vi "Reset old test Values (SubVI).vi"(8 "error in":errorcluster, 9 "Atr in":refnum<vi>, 11 "Test Paragraph":string) -> (0 "error out":errorcluster, 1 "Atr out":refnum<vi>, 2 "Line number":i32, 3 "Atr Out":string[][](array[string]))   [LabVIEW 2017]
uses:
  <vilib>/Utility/miscctls.llb/LVRowAndColumnTypeDef.ctl
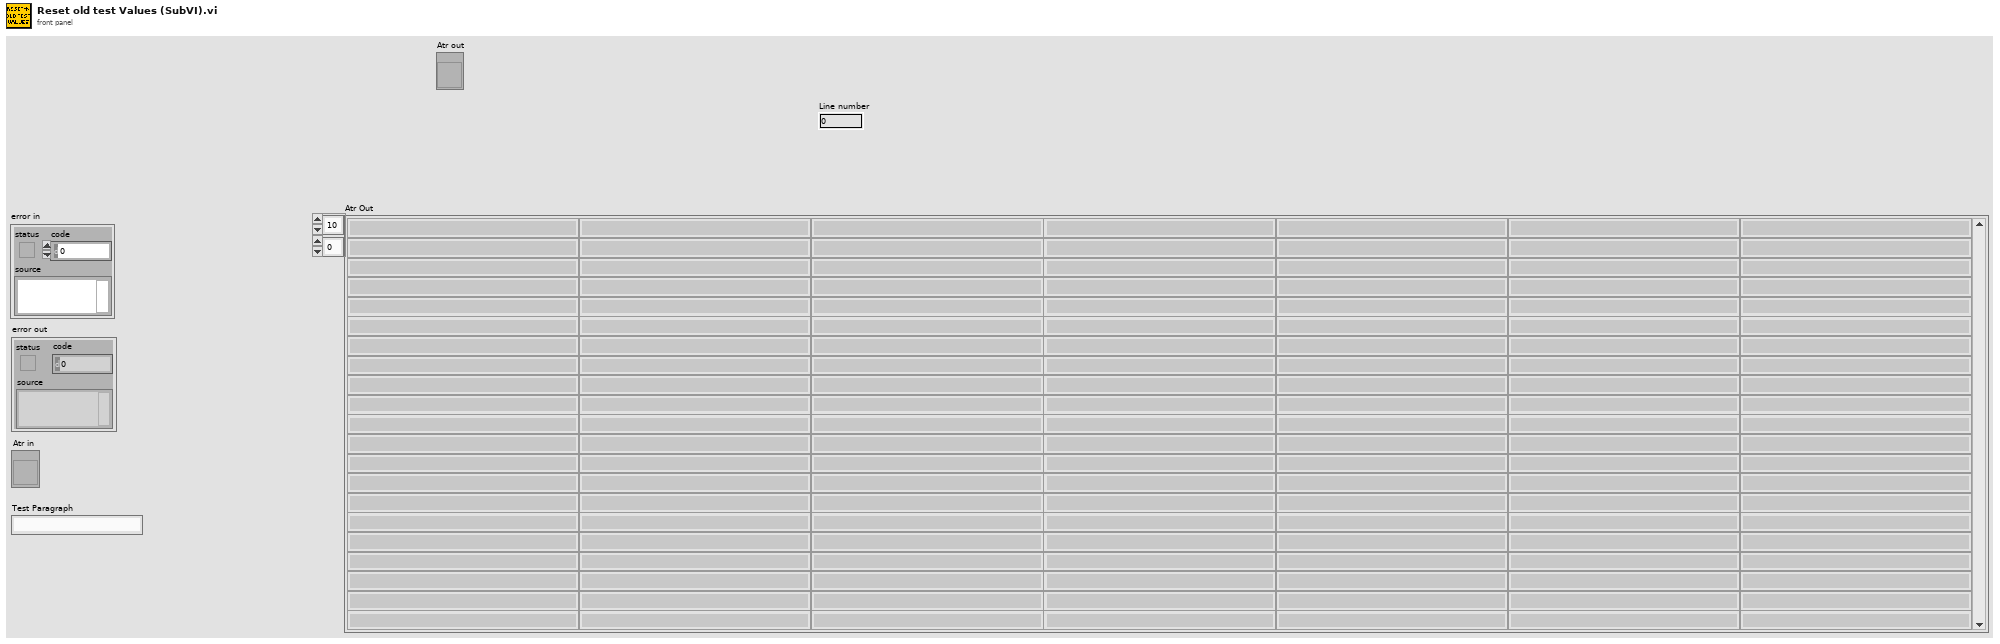
[diagram p1: front panel]
types:
  T1 = typedef "LVRowAndColumnTypeDef.ctl" = cluster{"Row":i32, "Column":i32}
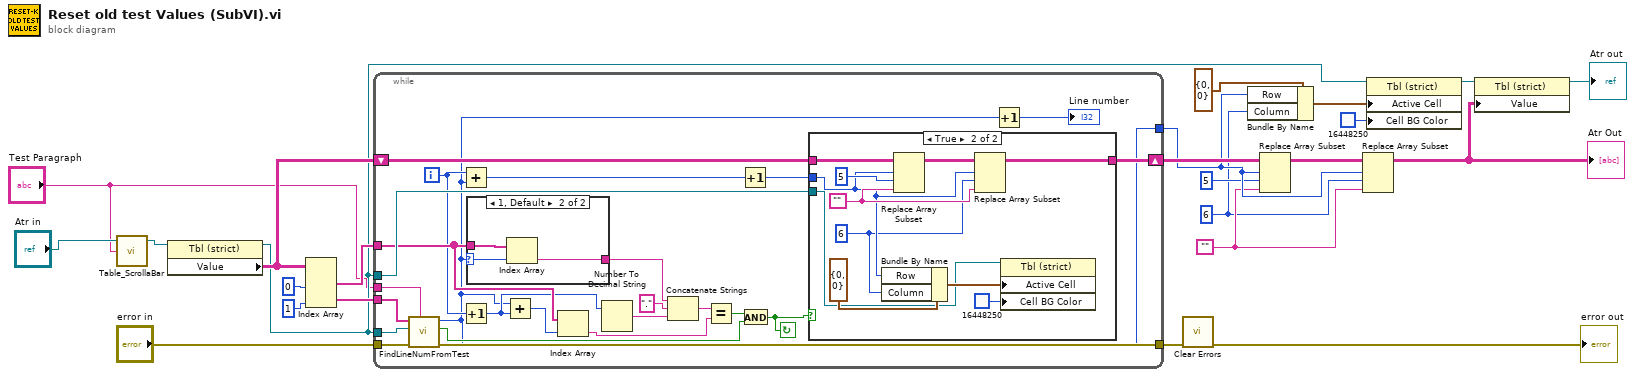
[diagram p0: block diagram]
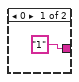
[diagram p2: hidden frame]
diagram:
  w11 = ""
  w8 = 6 ("disabled index (col)")
  n1 = call "Table_ScrollaBar.vi"("Line to focus"="Test Paragraph", "TableIn"="Atr in") -> ("Tableout"=w1:refnum<vi>)  [unwired: 2 in, 1 out]
  n2 = property class="Tbl (strict)"(reference=w1) -> (reference out=w15:refnum<vi>, "Value"=w17:string[][])  [unwired: 1 in, 1 out]
  n3 = Index Array(array=w17, index (col) #1=0 ("disabled index (col)"), index (col) #2=1 ("disabled index (col)")) -> (element #1=w18:string[], element #2=w20:string[])  [unwired: 2 in]
  n4 = while {
    tunnel: w20 -> [w48]
    tunnel: "Test Paragraph" -> [w41]
    tunnel: "error in" -> [w47]
    tunnel: [w46] -> w23
    shift-right: [w45] -> w16
    shift-left: w17 -> [w44]
    tunnel: w15 -> [w43]
    tunnel: w15 -> [w42]
    tunnel: w18 -> [w38]
    tunnel: [w26] -> w14
    i -> [w31]
    stop <- w35 continue-if-true
    n5 = call "FindLineNumFromTest.vi"("Test Paragraph"=w41, "error in"=w47, "TableIn"=w42, "Row Headers[]"=w48) -> ("error out"=w46:errorcluster, "Found"=w37:bool, "Line number"=w26:i32)  [unwired: 1 in, 1 out]
    n6 = Add(x=w31, y=w26) -> (x+y=w36:i32)
    n7 = Increment(x=w31) -> (x+1=w27:i32)
    n8 = case shown="1, Default" w26 {
      selector: w26 -> [_ w50]
      tunnel: w38 -> [_ w52]
      tunnel: ["1" w51] -> w29
      frame 0 {
      }
      frame 1, Default {
        n9 = Index Array(array=w52, index=w50) -> (element=w51:string)
      }
    }
    n10 = Add(x=w26, y=w27) -> (x+y=w32:i32)
    n11 = Index Array(array=w38, index=w32) -> (element=w34:string)
    n12 = Number To Decimal String(number=w27) -> (decimal integer string=w40:string)  [unwired: 1 in]
    n13 = Concatenate Strings(w29, "." ("string"), w40) -> (w33:string)
    n14 = Equal?(x=w33, y=w34) -> (x = y?=w30:bool)
    n15 = Increment(x=w36) -> (x+1=w28:i32)
    n16 = And(x=w30, y=w37) -> (x .and. y?=w35:bool)
    n17 = case shown="True" w35 {
      tunnel: [w53 w63] -> w45
      tunnel: w44 -> [w53 w62]
      tunnel: w28 -> [_ w57]
      tunnel: w43 -> [_ w54]
      frame False {
      }
      frame True {
        w60 = ""
        w56 = 6 ("disabled index (col)")
        n18 = Bundle By Name(cluster=T1 {"Row"=0, "Column"=0} ("Active Cell:Active Cell"), "Row"=w57, "Column"=w56) -> (w59:T1)
        n19 = Replace Array Subset(array=w62, new element=w60, index (row)=w57, index (col)=5 ("disabled index (col)")) -> (w64:string[][])
        n20 = Replace Array Subset(array=w64, new element=w60, index (row)=w57, index (col)=w56) -> (w63:string[][])
        n21 = property class="Tbl (strict)"(reference=w54, "Active Cell"=w59, "Cell BG Color"=u32 16448250) -> ()  [unwired: 1 in, 2 out]
      }
    }
    n22 = Increment(x=w26) -> (x+1=→"Line number":i32)
  }
  n23 = call <vilib>:"Clear Errors.vi"("error in (no error)"=w23) -> ("error out"=→"error out":errorcluster)  [unwired: 5 in, 1 out]
  n24 = Bundle By Name(cluster=T1 {"Row"=0, "Column"=0} ("Active Cell:Active Cell"), "Row"=w14, "Column"=w8) -> (w10:T1)
  n25 = Replace Array Subset(array=w16, new element=w11, index (row)=w14, index (col)=5 ("disabled index (col)")) -> (w13:string[][])
  n26 = Replace Array Subset(array=w13, new element=w11, index (row)=w14, index (col)=w8) -> (w4:string[][])
  "Atr Out" <- w4
  n27 = property class="Tbl (strict)"(reference=w15, "Active Cell"=w10, "Cell BG Color"=u32 16448250) -> (reference out=w6:refnum<vi>)  [unwired: 1 in, 1 out]
  n28 = property class="Tbl (strict)"(reference=w6, "Value"=w4) -> (reference out=→"Atr out":refnum<vi>)  [unwired: 1 in, 1 out]
